vi "SSL_new.vi"(8 "error in (no error)":errorcluster, 11 "SSL-Context in":refnum<class "SSL-Context.lvclass">) -> (0 "error out":errorcluster, 2 "SSL out":refnum<class "SSL.lvclass">, 3 "SSL-Context out":refnum<class "SSL-Context.lvclass">)   [LabVIEW 2013, in "OpenSSL Socket.lvlib" / "SSL-Context.lvclass"]
uses:
  SSL-Context.lvclass
  SSL/SSL.lvclass
  SSL-Lib/SSL-Lib.lvclass/SSL-Lib.ctl
  SSL-Context.lvclass/SSL-Context.ctl
  SSL/SSL.lvclass/SSL.ctl
  SSL-Lib/Read SSL Library Path.vi
  Read Handle.vi
  SSL/Write Handle.vi
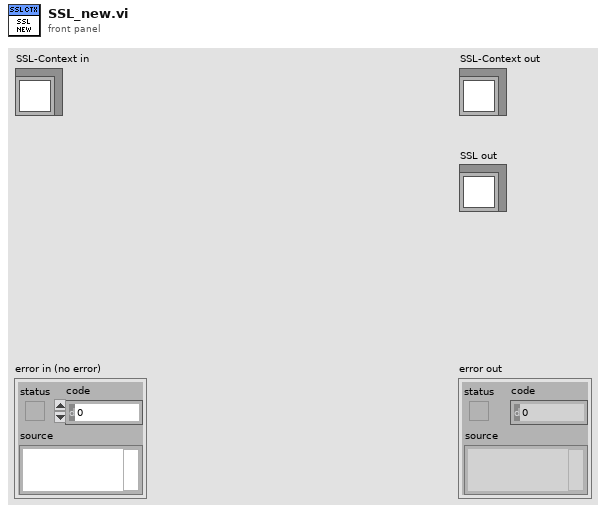
[diagram p1: front panel]
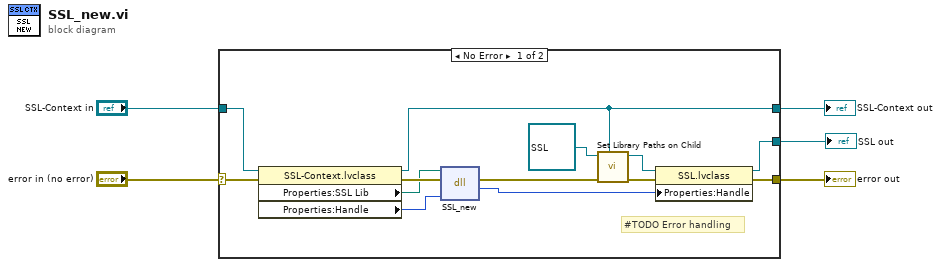
[diagram p0: block diagram]
diagram:
  n1 = case shown="No Error" "error in (no error)" {
    selector: "error in (no error)" -> [w18 w20]
    tunnel: [w10 w20] -> w4
    tunnel: [w11 w19] -> w2
    tunnel: "SSL-Context in" -> [w16 w19]
    tunnel: [w6 _] -> w1
    frame No Error {
      # "#TODO Error handling"
      n2 = property class="SSL-Context.lvclass"(reference=w16, error in=w18) -> (reference out=w11:refnum<class "SSL-Context.lvclass">, error out=w17:errorcluster, "Properties:SSL Lib"=w15:path, "Properties:Handle"=w14:u64)
      n3 = dll-call lib="C:/Program Files (x86)/National Instruments/Shared/nissl/NIssleay32.dll" fn="SSL_new"(path in=w15, error in=w17, "SSL_CTX"=w14) -> (error out=w13:errorcluster, "SSL"=w7:u64)  [unwired: 2 in, 1 out]
      n4 = call-dynamic "Set Library Paths on Child.vi"(7:"SSL-Lib in"=w11, "error in (no error)"=w13, 11:"SSL-Lib in"=refnum<class "SSL.lvclass"> refnum ("SSL_Lib.lvlib:SSL.lvclass")) -> ("error out"=w9:errorcluster, "SSL-Lib out"=w8:refnum<class "SSL.lvclass">)  [unwired: 7 in]
      n5 = property class="SSL.lvclass"(reference=w8, error in=w9, "Properties:Handle"=w7) -> (reference out=w6:refnum<class "SSL.lvclass">, error out=w10:errorcluster)
    }
    frame Error {
    }
  }
  "error out" <- w4
  "SSL-Context out" <- w2
  "SSL out" <- w1
